vi "Idle.vi"(8 "error in":errorcluster, 11 "Plugin_Controller in":refnum<class "Plugin_Controller.lvclass">) -> (0 "error out":errorcluster, 3 "Plugin_Controller out":refnum<class "Plugin_Controller.lvclass">)   [LabVIEW 2020, in "Plugin.lvlib" / "Plugin_Controller.lvclass"]
doc: "This VI will Clears the buffer until all other configured Plugins are completed executing their Initialize states. This process will ensure synchronized start for all Plugins."
uses:
  Plugin_Controller.lvclass
  C:/SVN_LabSys/labsys_lvcode/LabSys_SourceCode/builds/Libraries/LabSys Framework.lvlibp/Data Node/Data Node/Data Node.lvclass
  C:/SVN_LabSys/labsys_lvcode/LabSys_SourceCode/builds/Libraries/LabSys Framework.lvlibp/Configurable Data Node/Configurable Data Node/Configurable Data Node.lvclass
  Plugin_Controller.lvclass/Plugin_Controller.ctl
  builds/Libraries/LabSys Framework.lvlibp/Data Node/Data Node/Read Error Manager.vi
  builds/Libraries/LabSys Framework.lvlibp/Configurable Data Node/Configurable Data Node/Read Module Configuration.vi
  builds/Libraries/LabSys Framework.lvlibp/Configuration Storage/Module Configuration/Read Module Name.vi
  builds/Libraries/LabSys Framework.lvlibp/Error Manager/Error Manager/Error Manager.lvclass
  builds/Libraries/LabSys Framework.lvlibp/Configuration Storage/Module Configuration/Module Configuration.lvclass
  Plugin_Driver/Plugin_Driver.lvclass
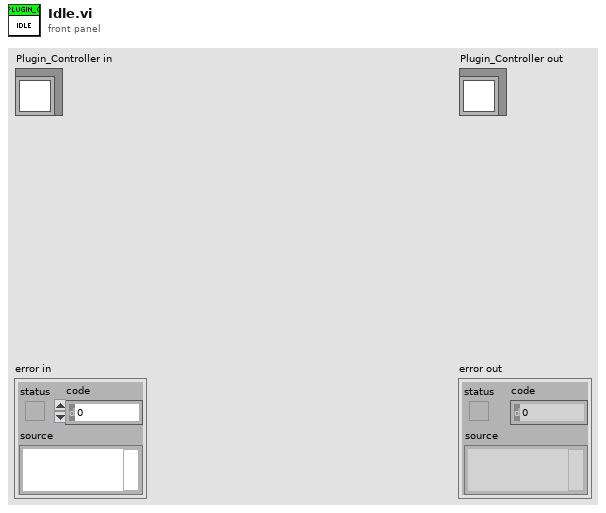
[diagram p1: front panel]
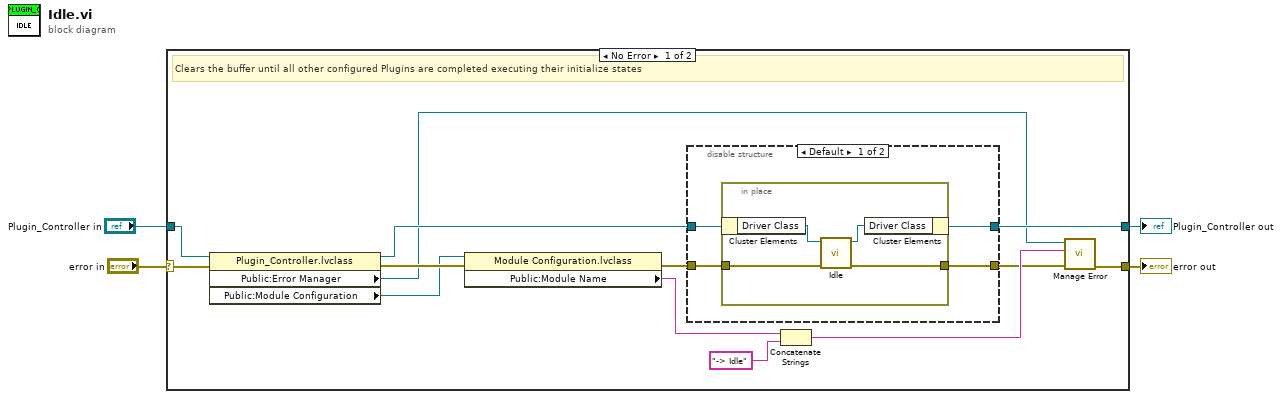
[diagram p0: block diagram]
diagram:
  n1 = case shown="No Error" "error in" {
    selector: "error in" -> [w15 w29]
    tunnel: [w9 w29] -> w3
    tunnel: [w13 w28] -> w1
    tunnel: "Plugin_Controller in" -> [w14 w28]
    frame No Error {
      # "Clears the buffer until all other configured Plugins are completed executing their initialize states"
      n2 = property class="Plugin_Controller.lvclass"(reference=w14, error in=w15) -> (reference out=w17:refnum<class "Plugin_Controller.lvclass">, error out=w16:errorcluster, "Public:Error Manager"=w11:refnum<data-value>, "Public:Module Configuration"=w6:refnum<class "Module Configuration.lvclass">)
      n3 = property class="Module Configuration.lvclass"(reference=w6, error in=w16) -> (error out=w7:errorcluster, "Public:Module Name"=w5:string)  [unwired: 1 out]
      n4 = disable-structure shown="Default" {
        disable-tunnel: [w21 w27] -> w13
        disable-tunnel: [w20 w26] -> w8
        disable-tunnel: w17 -> [w19 w27]
        disable-tunnel: w7 -> [w18 w26]
        frame condition #0 (active) {
          n5 = in-place {
            in-place-border: [w22] -> w20
            in-place-border: w18 -> [w23]
            n6 = in-place-cluster #1(w19) -> ("Driver Class"=w25:refnum<class "Plugin_Driver.lvclass">)
            n7 = call "Idle.vi"("error in"=w23, "Plugin_Driver in"=w25) -> ("error out"=w22:errorcluster, "Plugin_Driver out"=w24:refnum<class "Plugin_Driver.lvclass">)  [unwired: 8 in]
            n8 = in-place-cluster #1("Driver Class"=w24) -> (w21:refnum<class "Plugin_Controller.lvclass">)
          }
        }
        frame condition #1 {
        }
      }
      n9 = Concatenate Strings(w5, "-> Idle" ("string")) -> (w12:string)
      n10 = call "Manage Error.vi"("error in (no error)"=w8, "Error Location"=w12, "Error Manager in"=w11) -> ("error out"=w9:errorcluster)  [unwired: 7 in, 1 out]
    }
    frame Error {
    }
  }
  "error out" <- w3
  "Plugin_Controller out" <- w1
